vi "add_tail.vi"(8 "error in (no error)":errorcluster, 10 "data":variant, 11 "IList in":refnum<class "IList.lvclass">) -> (0 "error out":errorcluster, 3 "IList out":refnum<class "IList.lvclass">)   [LabVIEW 2021, in "IList.lvclass"]
uses:
  IList.lvclass
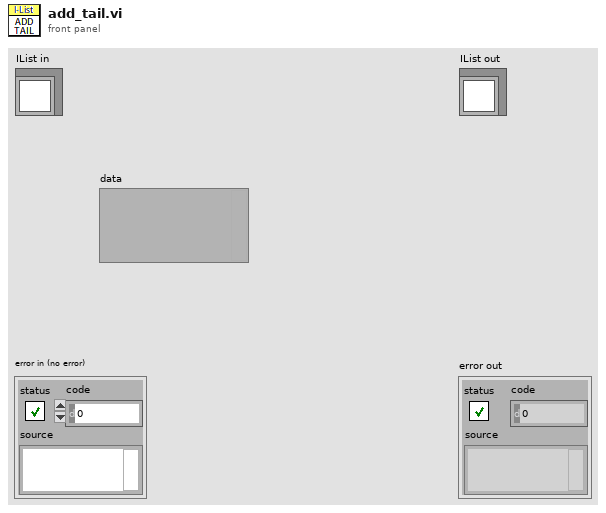
[diagram p1: front panel]
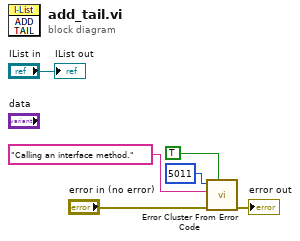
[diagram p0: block diagram]
diagram:
  n1 = call <vilib>:"Error Cluster From Error Code.vi"("show call chain? (False)"=TRUE, "error in (no error)"="error in (no error)", "error message (\"\")"="Calling an interface method." ("error message (\"\")"), "error code (0)"=5011) -> ("error out"=→"error out":errorcluster)  [unwired: 5 in]
  "IList out" <- "IList in"
